vi "PFI-28000-Base_Query.vi"(0 "PFI-28000-Base in":refnum<class "PFI-28000-Base.lvclass">, 5 "Command":string, 11 "error in (no error)":errorcluster) -> (4 "PFI-28000-Base out":refnum<class "PFI-28000-Base.lvclass">, 6 "Response":string, 8 "Timed Out":bool, 15 "error out":errorcluster)   [LabVIEW 2017, in "PFI-28000-Base.lvclass"]
uses:
  PFI-28000-Base.lvclass
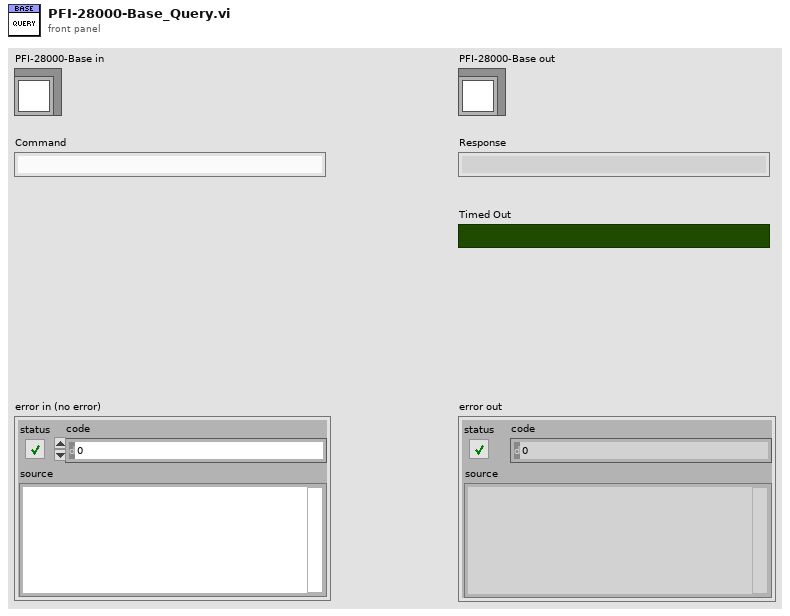
[diagram p1: front panel]
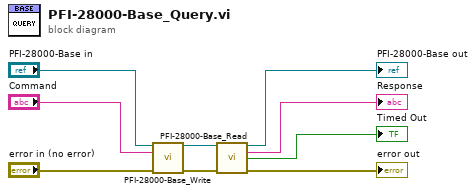
[diagram p0: block diagram]
diagram:
  n1 = call-dynamic "PFI-28000-Base_Write.vi"("PFI-28000-Base in"="PFI-28000-Base in", "Command"="Command", "error in (no error)"="error in (no error)") -> ("PFI-28000-Base out"=w9:refnum<class "PFI-28000-Base.lvclass">, "error out"=w8:errorcluster)  [unwired: 11 in]
  n2 = call-dynamic "PFI-28000-Base_Read.vi"("PFI-28000-Base in"=w9, "error in (no error)"=w8) -> ("PFI-28000-Base out"=→"PFI-28000-Base out":refnum<class "PFI-28000-Base.lvclass">, "Response"=→"Response":string, "Timed Out"=→"Timed Out":bool, "error out"=→"error out":errorcluster)  [unwired: 10 in]
